vi "practica4.vi"() -> ()   [LabVIEW 2014]
uses:
  <vilib>/MakerHub/LINX/Public/Peripherals/Analog/Analog Read 1 Chan.vi
  <vilib>/MakerHub/LINX/Public/Peripherals/Digital/Digital Write 1 Chan.vi
  <vilib>/MakerHub/LINX/Public/Peripherals/Analog/Analog Read N Chans.vi
  <vilib>/MakerHub/LINX/Public/Peripherals/Digital/Digital Write N Chans.vi
  <vilib>/MakerHub/LINX/Private/Local IO/LinxAnalogRead.vi
  <vilib>/MakerHub/LINX/Public/Utilities/Check Channel.vi
  <vilib>/MakerHub/LINX/Private/Local IO/LinxDigitalWrite.vi
  <vilib>/MakerHub/LINX/Public/Utilities/Open Serial.vi
  <vilib>/MakerHub/LINX/Private/Utilties/Generate Error.vi
  <vilib>/MakerHub/LINX/LMH-LINX.lvlib
panel:
  in  "Stop Button":bool
  in  "DO Channel Led3":u8
  in  "DO Channel Led2":u8
  in  "D0 Channel Led1":u8
  out "Voltage":dbl
  out "Boolean 3":bool
  out "Boolean 2":bool
  out "Boolean":bool
  in  "Analog Channel fotorresistencia":u8
  in  "Serial Port":refnum<visa-resource-name>="N/A"
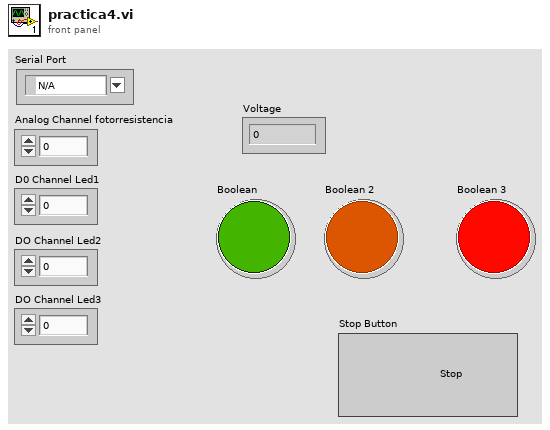
[diagram p1: front panel]
types:
  T1 = typedef "LMH-LINX.lvlib/LINX Ref.ctl" = cluster{"IO":T2, "Interface":T3, "LINX Device Config":T4}
  T2 = typedef "LMH-LINX.lvlib/Platform.ctl" = enum16{"Remote", "Local"}
  T3 = typedef "LMH-LINX.lvlib/Interface.ctl" = enum16{"Serial", "TCP"}
  T4 = typedef "LMH-LINX.lvlib/Device.lvlib/LINX Device Config.ctl" = cluster{"Interface":T3, "COM Port":refnum<visa-resource-name>, "TCP Configuration":T5, "Device Family":u8, "Device ID":u8, "Device Name":string, "TCP Ref":refnum<k5>, "Channels":T6}
  T5 = typedef "LMH-LINX.lvlib/Device.lvlib/TCP Config.ctl" = cluster{"IP Address":string, "Port":u16}
  T6 = typedef "LMH-LINX.lvlib/Channels.ctl" = cluster{"DI":u8[], "DO":u8[], "AI":u8[], "AO":u8[], "PWM":u8[], "QE":u8[], "UART":u8[], "I2C 2":u8[], "SPI":u8[], "CAN":u8[], "Servo":u8[], "AI Ref (V)":dbl, "AI Resolution (Bits)":u8, "AO Ref (V)":dbl, "AO Resolution (Bits)":u8}
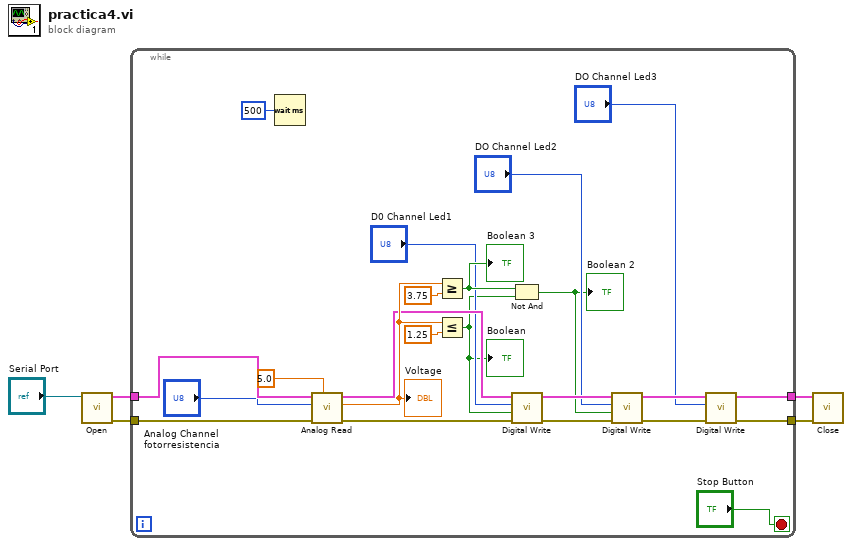
[diagram p0: block diagram]
diagram:
  n1 = call-poly <vilib>:"Open.vi"("Serial Port"="Serial Port") -> ("Error Out"=w3:errorcluster, "LINX Resource"=w4:T1)  [unwired: 8 in, 1 out]
  n2 = while {
    tunnel: w4 -> [w28]
    tunnel: w3 -> [w27]
    tunnel: [w8] -> w2
    tunnel: [w7] -> w1
    stop <- "Stop Button" stop-if-true
    n3 = Wait (ms)(milliseconds to wait=u32 500) -> ()  [unwired: 1 out]
    n4 = call-poly <vilib>:"Analog Read.vi"("Analog Ref Override (V)"=5.0, "Error In"=w27, "Analog Channel"="Analog Channel fotorresistencia", "LINX Resource"=w28) -> ("Error Out"=w19:errorcluster, "Voltage"=w23:dbl, "LINX Resource"=w20:T1)  [unwired: 4 in, 1 out]
    "Voltage" <- w23
    n5 = Greater Or Equal?(x=w23, y=3.75) -> (x >= y?=w21:bool)
    "Boolean 3" <- w21
    n6 = Less Or Equal?(x=w23, y=1.25) -> (x <= y?=w17:bool)
    "Boolean" <- w17
    n7 = Not And(1:w17, 2:w21) -> (0:w13:bool)
    "Boolean 2" <- w13
    n8 = call-poly <vilib>:"Digital Write.vi"("Error In"=w19, "Output Value"=w17, "DO Channel"="D0 Channel Led1", "LINX Resource"=w20) -> ("Error Out"=w15:errorcluster, "LINX Resource"=w16:T1)  [unwired: 6 in]
    n9 = call-poly <vilib>:"Digital Write.vi"("Error In"=w15, "Output Value"=w13, "DO Channel"="DO Channel Led2", "LINX Resource"=w16) -> ("Error Out"=w11:errorcluster, "LINX Resource"=w12:T1)  [unwired: 6 in]
    n10 = call-poly <vilib>:"Digital Write.vi"("Error In"=w11, "DO Channel"="DO Channel Led3", "LINX Resource"=w12) -> ("Error Out"=w7:errorcluster, "LINX Resource"=w8:T1)  [unwired: 7 in]
  }
  n11 = call <vilib>:"Close.vi"("Error In"=w1, "LINX Resource"=w2) -> ()  [unwired: 9 in, 1 out]
